vi "Enqueue.vi"(8 "error in (no error)":errorcluster, 10 "State":string, 11 "Masterv2 in":refnum<class "Masterv2.lvclass">) -> (0 "error out":errorcluster, 3 "Masterv2 out":refnum<class "Masterv2.lvclass">)   [LabVIEW 2014, in "Main Libraryv2.lvlib" / "Masterv2.lvclass"]
uses:
  Master/Masterv2.lvclass
panel:
  in  "Data":variant
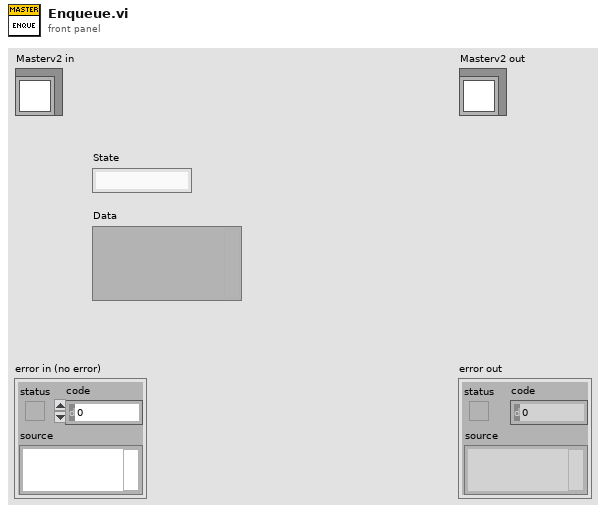
[diagram p1: front panel]
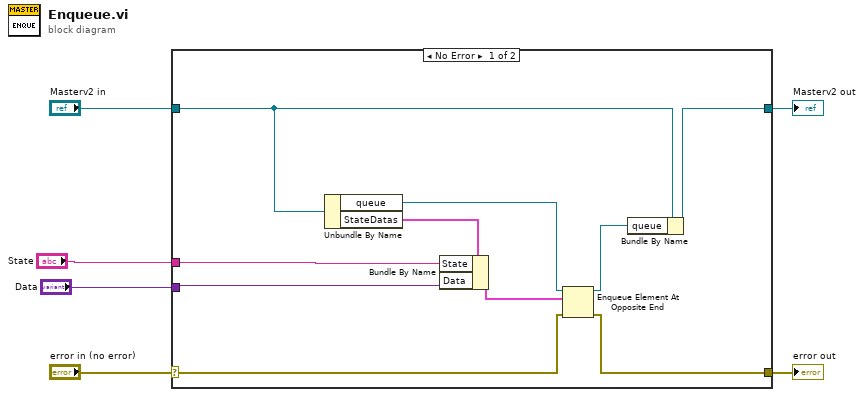
[diagram p0: block diagram]
diagram:
  n1 = case shown="No Error" "error in (no error)" {
    selector: "error in (no error)" -> [w8 w18]
    tunnel: [w7 w18] -> w5
    tunnel: [w9 w17] -> w3
    tunnel: "Masterv2 in" -> [w10 w17]
    tunnel: "State" -> [w16 _]
    tunnel: "Data" -> [w15 _]
    frame No Error {
      n2 = Unbundle By Name(w10) -> ("queue"=w12:refnum<queue>, "StateDatas"=w14:cluster{"State":string, "Data":variant})
      n3 = Bundle By Name(cluster=w14, "State"=w16, "Data"=w15) -> (w13:cluster{"State":string, "Data":variant})
      n4 = Enqueue Element At Opposite End(queue=w12, element=w13, error in (no error)=w8) -> (queue out=w11:refnum<queue>, error out=w7:errorcluster)  [unwired: 1 in, 1 out]
      n5 = Bundle By Name(cluster=w10, "queue"=w11) -> (w9:refnum<class "Masterv2.lvclass">)
    }
    frame Error {
    }
  }
  "error out" <- w5
  "Masterv2 out" <- w3
